vi "AlGaInPAs_prep_run_cont_dil_v17.vi"(2 "Debug Mode":bool, 3 "Elapsed Time(s)":dbl, 4 "State":enum16{"Edit", "Start", "Run", "End", "Idle"}(ring), 5 "Argument List In":string[](array[string])) -> (0 "Status Out":string, 1 "Argument List Out":string[](array[string]))   [LabVIEW 2011]
panel:
  out "GAMFC3 var":dbl=100.0 caption="R3 (0-1000 sscm)" format="%.1f"
  out "GAMFC2 var":dbl=10.0 caption="R2 (0-100 sscm)" format="%.2f"
  out "GAMFC1 var":dbl=1.0 caption="R1 (0-10 sscm)" format="%.2f"
  out "Ga Flow var":dbl=1.0 caption="Ga Flow (0-10 sscm)" format="%.4f"
  out "Prep-In var":bool
  out "Prep-Ga var":bool
  out "Prep-Al var":bool
  out "Prep-P var":bool
  out "Prep-As var":bool
  out "prep_done":bool
  out "run started":bool
  out "first":bool=TRUE
  out "total time":dbl
  out "is OK?":bool
  out "AsH3?":bool
  out "PH3?":bool
  out "In?":bool
  out "Ga?":bool
  out "Al?":bool
  in  "Prep As":bool caption="Pre-run"
  in  "Prep P":bool caption="Pre-run"
  in  "Prep In":bool caption="Pre-run"
  in  "prep_time":dbl caption="pre-run time (s)"
  in  "Prep Al":bool caption="Pre-run"
  in  "Run As":bool caption="Run"
  in  "AsH3 Flow":dbl caption="AsH3 Flow (0-10 sccm)" format="%.2f"
  in  "P Flow":dbl caption="P Flow (0-100 sccm)" format="%.2f"
  in  "Run P":bool caption="Run"
  in  "In Flow":dbl caption="In Flow (0-100 sscm)" format="%.2f"
  in  "Run In":bool caption="Run"
  in  "Run Al":bool caption="Run"
  in  "Al Flow":dbl caption="Al Flow (0-100 sscm)" format="%.2f"
  in  "Cancel":bool
  in  "OK":bool
  out "tTotal(s) 2":dbl
  in  "Ga Tab Control":enum32{"Page 1", "Page 2", "Page 3"}(tab)
  in  "Ga Dilution":bool caption="Dilute"
  in  "Run Ga":bool caption="Run"
  in  "Prep Ga":bool caption="Pre-run"
  out "Ga Flow val":dbl=1.0 caption="Ga Flow (0-10 sscm)" format="%.4f"
  in  "Ga Flow set":dbl=1.0 caption="Ga Flow (0-10 sscm)" format="%.4f"
  out "GAMFC1 val":dbl=1.0 caption="R1 (0-10 sscm)" format="%.4f"
  out "GAMFC3 val":dbl=100.0 caption="R3 (0-1000 sscm)" format="%.1f"
  out "GAMFC2 val":dbl=10.0 caption="R2 (0-100 sscm)" format="%.2f"
  in  "GAMFC1 set":dbl=1.0 caption="R1 (0-10 sscm)" format="%.2f"
  in  "GAMFC2 set":dbl=10.0 caption="R2 (0-100 sscm)" format="%.2f"
  in  "GAMFC3 set":dbl=100.0 caption="R3 (0-1000 sscm)" format="%.1f"
  in  "Ga Calculated":u16(ring)=1 caption="Calculated" items=["Ga flow", "MFC1", "MFC2", "MFC3"]
  # "Add pre-run time to run time in editor."
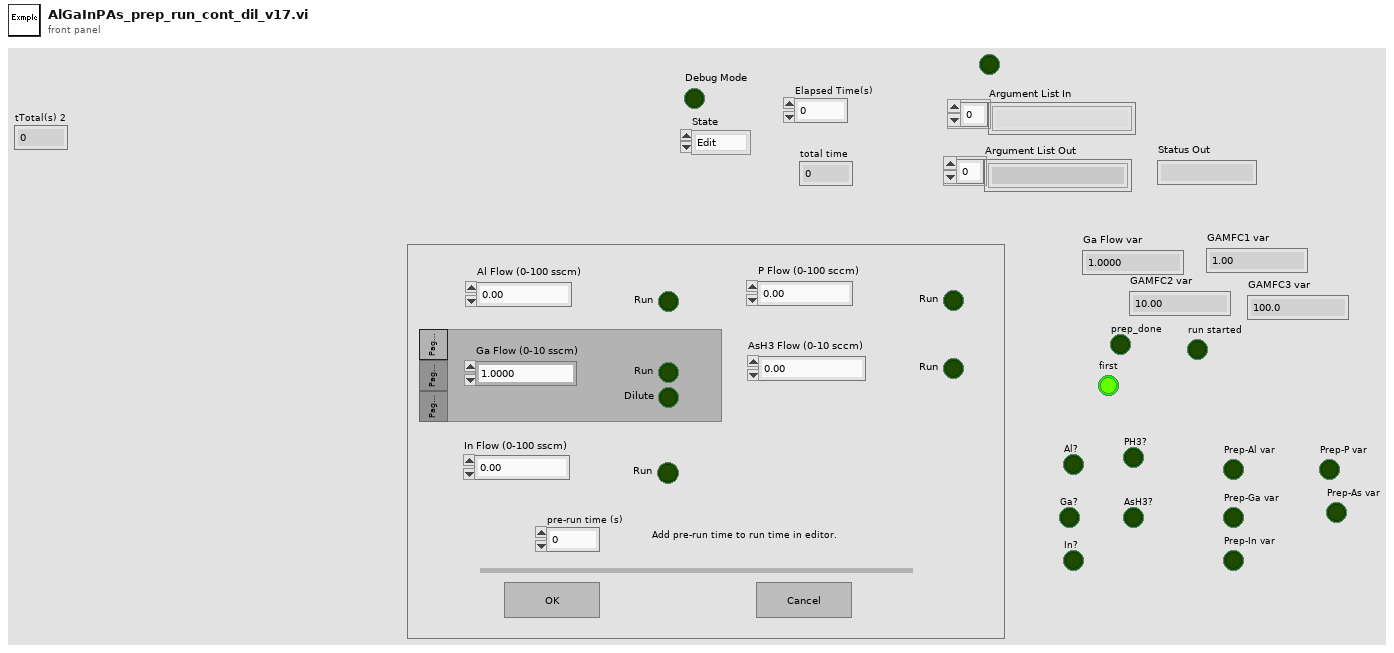
[diagram p1: front panel]
types:
  T1 = enum16{"Discrete", "Continuous", "Instantaneous", "Finite"}
  T2 = enum32{"Invalid", "Default", "Floating", "Floating/Auto-Hide", "Modal"}
  T3 = cluster{"Ga val":bool, "MFC1 val":bool, "MFC2 val":bool, "MFC3 val":bool, "Ga set":bool, "MFC1 set":bool, "MFC2 set":bool, "MFC3 set":bool}
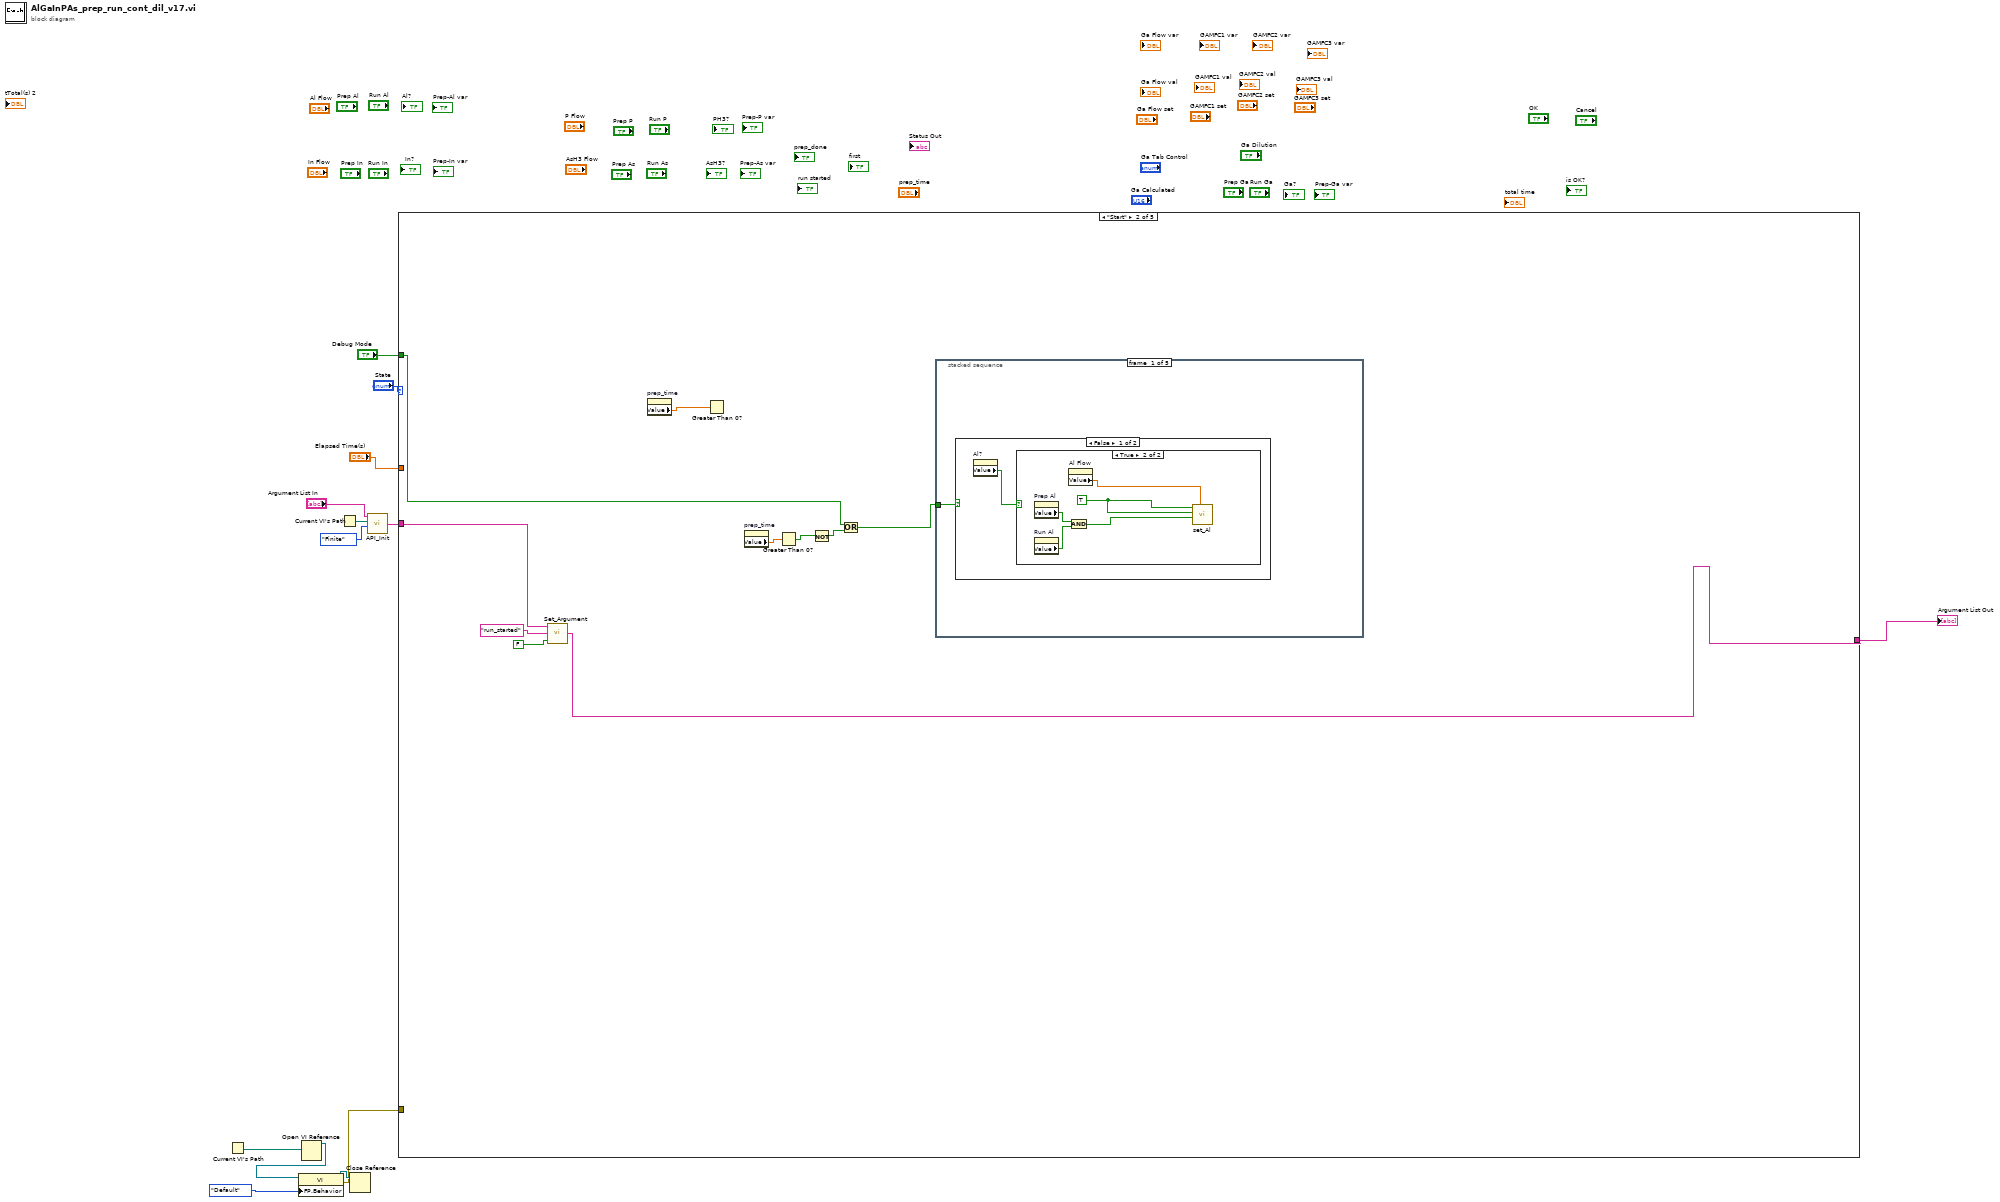
[diagram p0: block diagram]
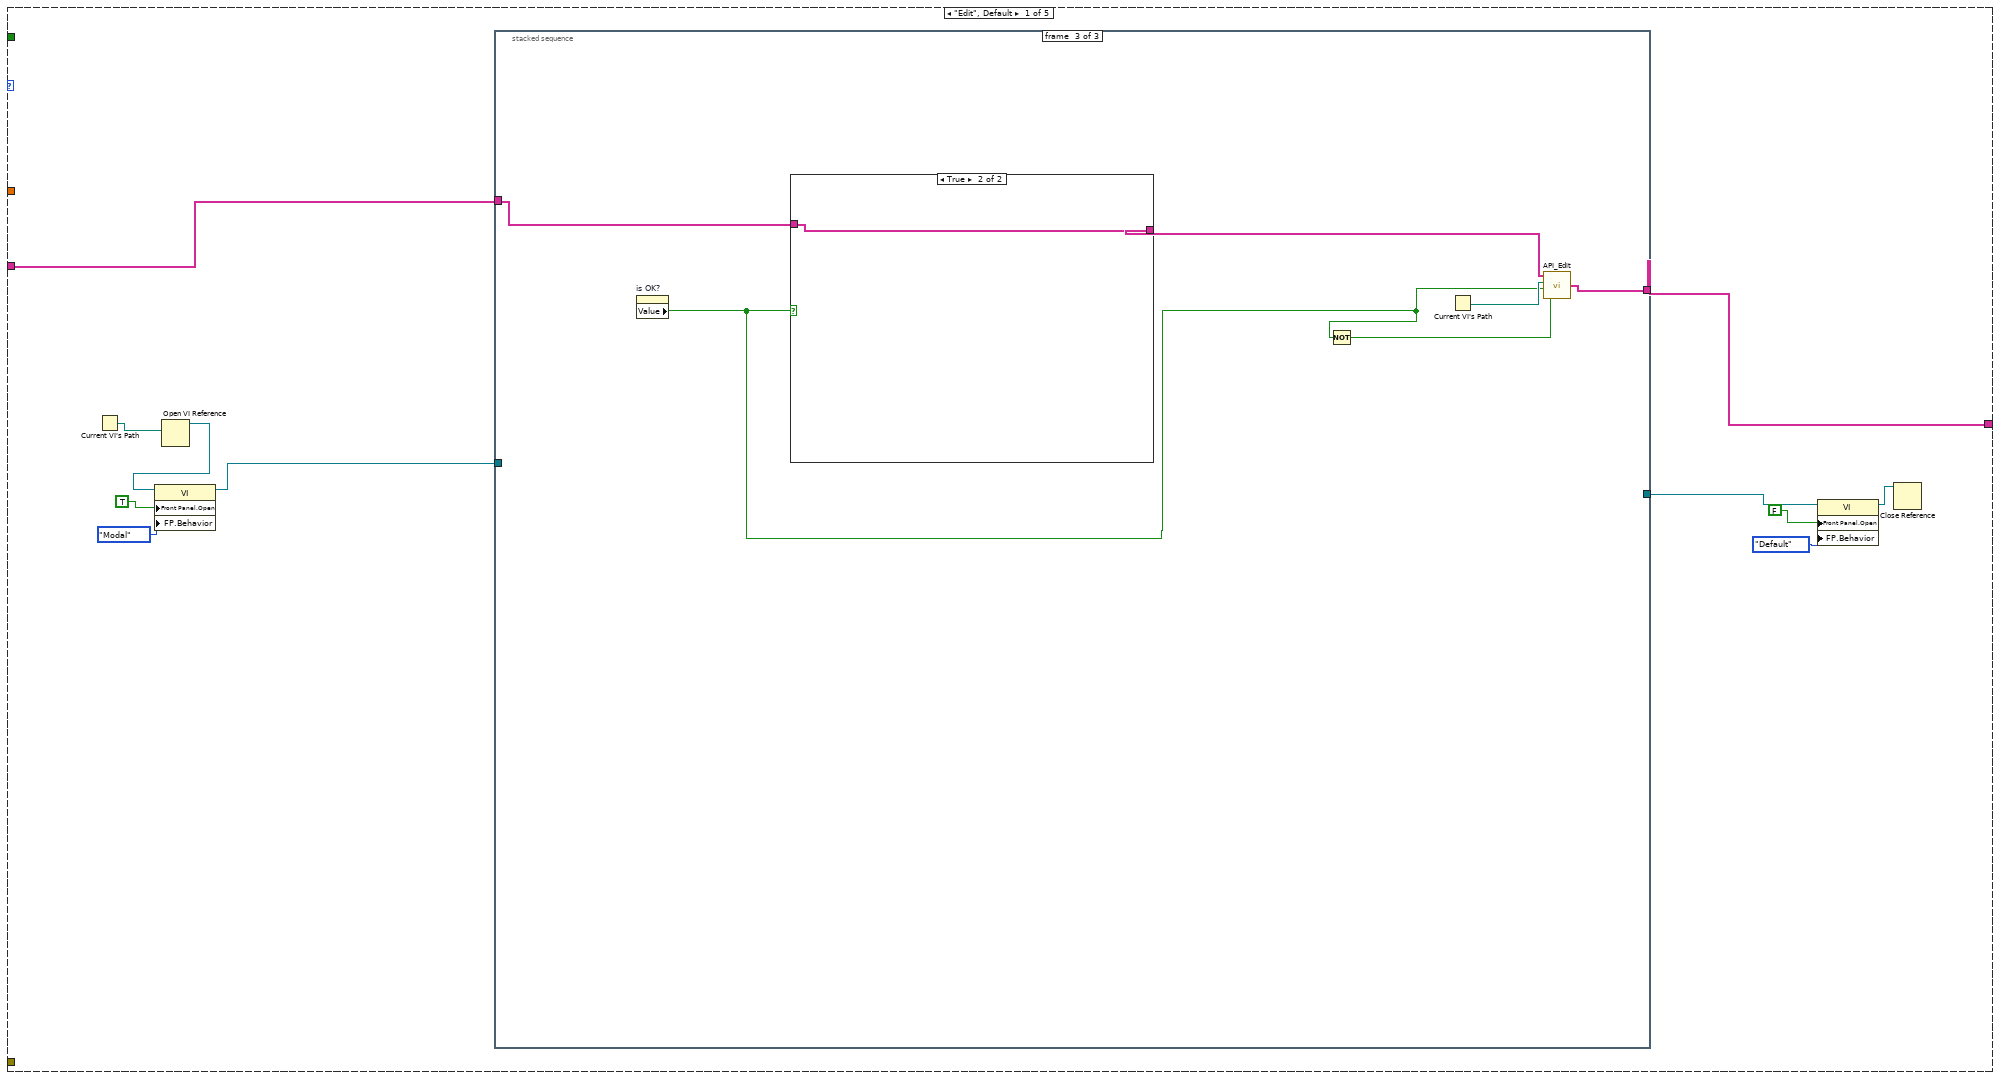
[diagram p2: hidden frame]
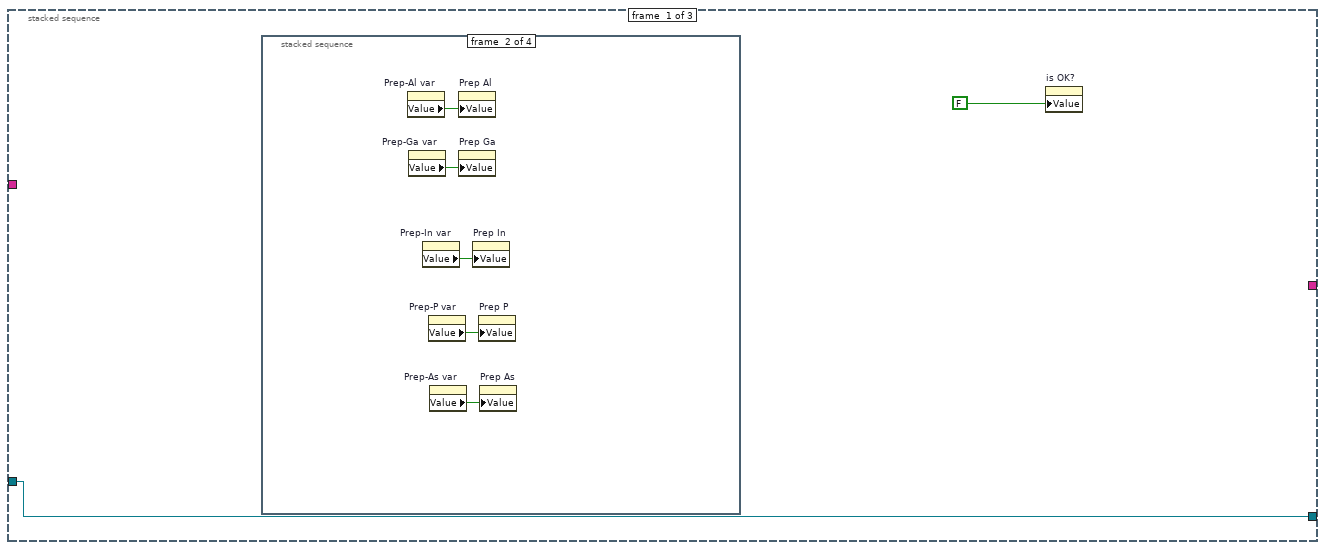
[diagram p3: hidden frame]
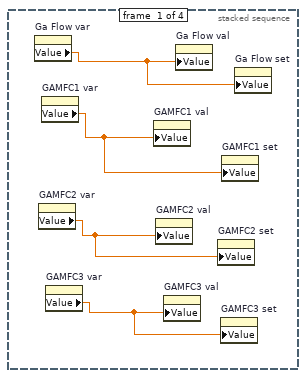
[diagram p4: hidden frame]
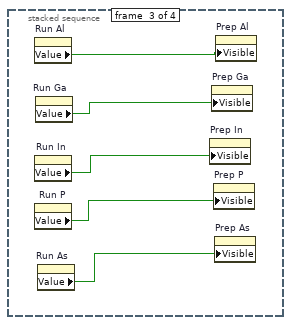
[diagram p5: hidden frame]
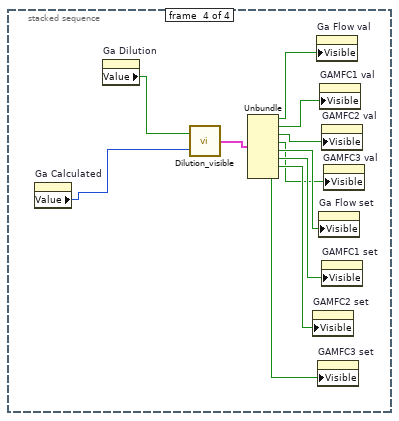
[diagram p6: hidden frame]
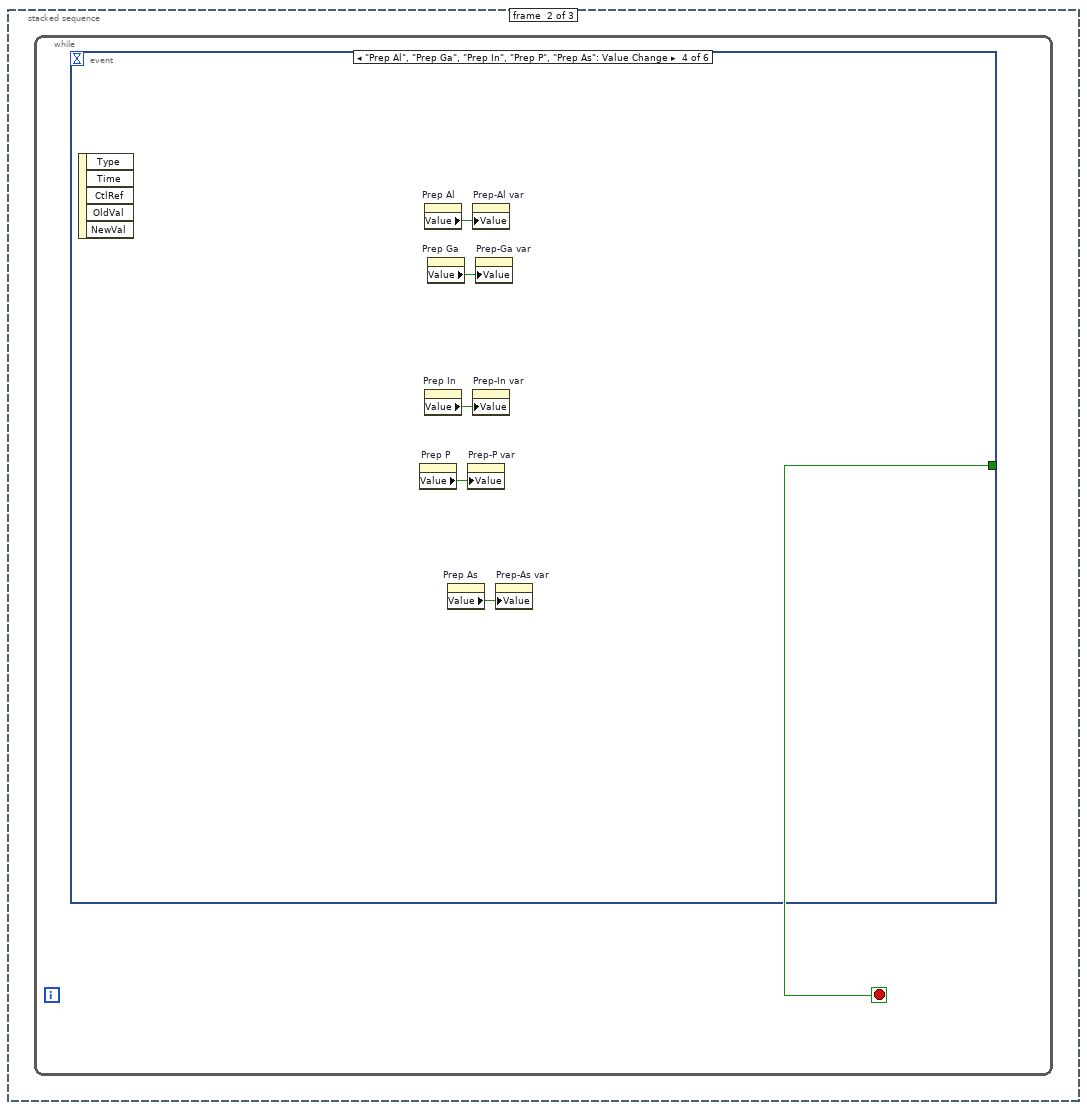
[diagram p7: hidden frame]
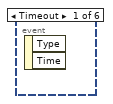
[diagram p8: hidden frame]
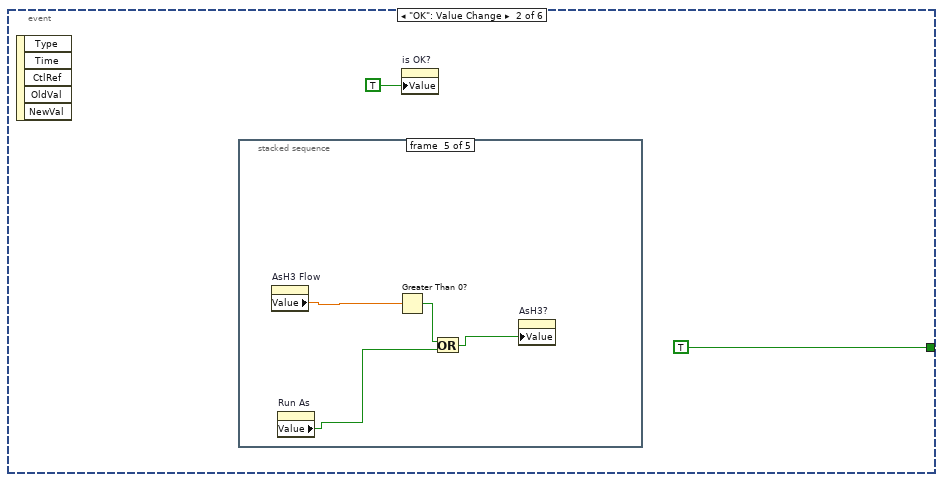
[diagram p9: hidden frame]
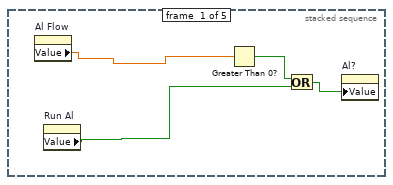
[diagram p10: hidden frame]
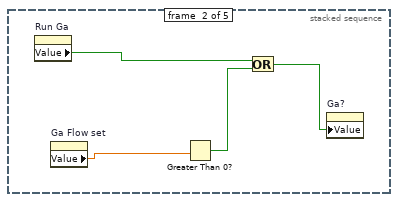
[diagram p11: hidden frame]
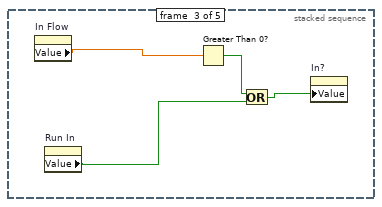
[diagram p12: hidden frame]
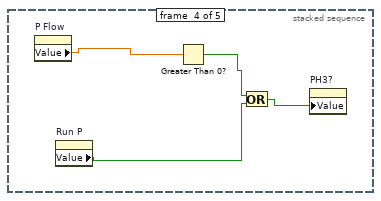
[diagram p13: hidden frame]
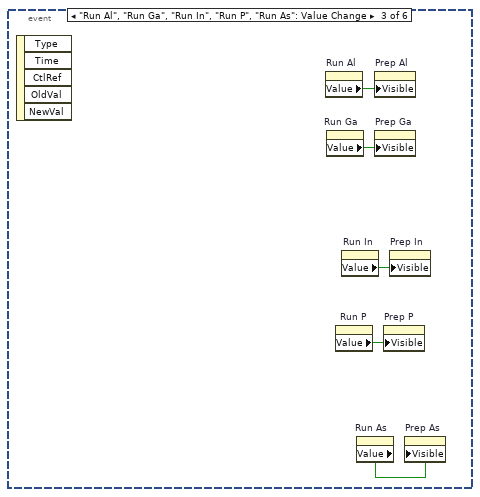
[diagram p14: hidden frame]
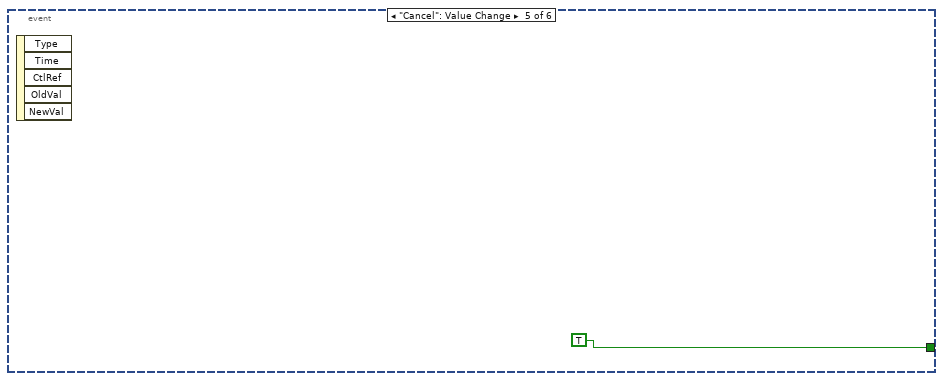
[diagram p15: hidden frame]
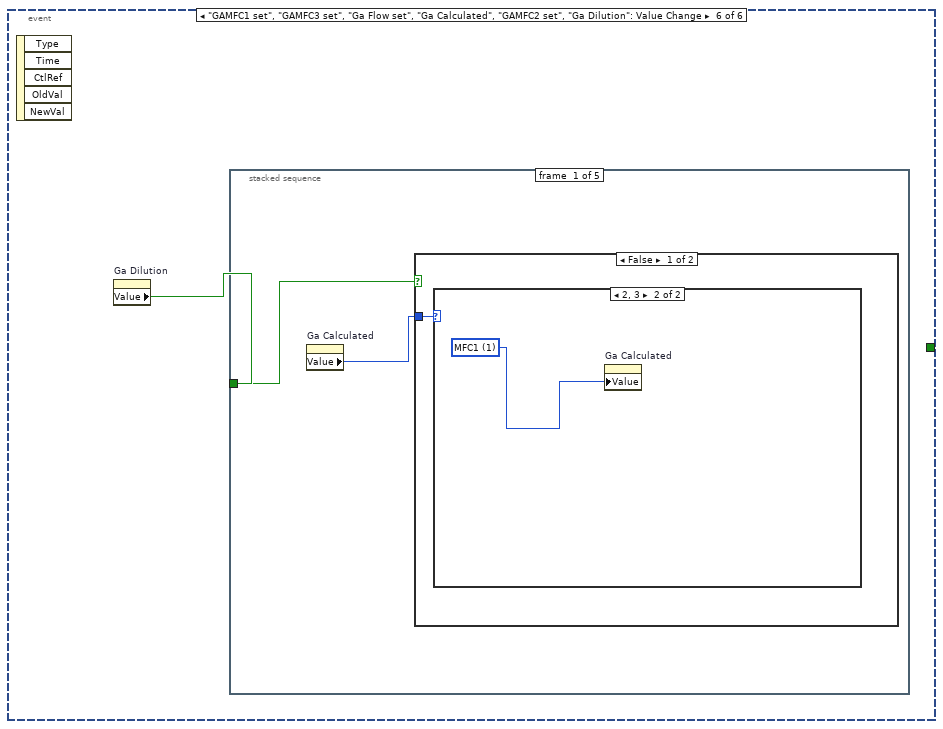
[diagram p16: hidden frame]
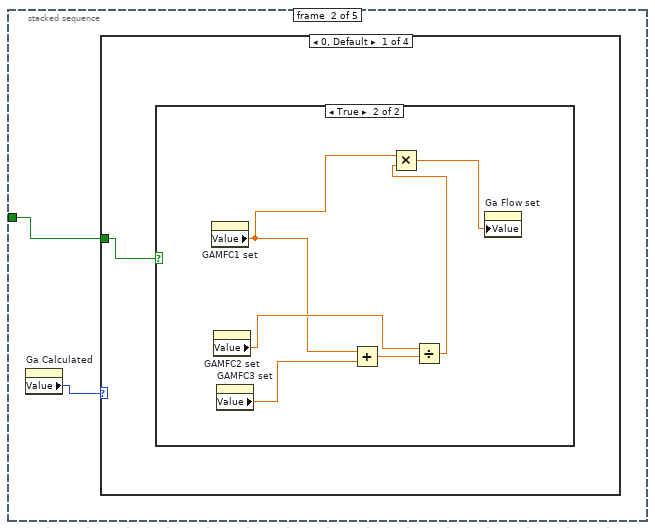
[diagram p19: hidden frame]
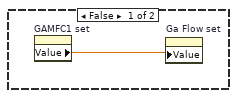
[diagram p20: hidden frame]
diagram:
  n1 = Current VI's Path() -> (path=w9:path)
  n2 = Open VI Reference(vi path=w9) -> (vi reference=w8:refnum<vi>)  [unwired: 1 in, 5 out]
  n3 = property class="VI"(reference=w8, "FP.Behavior"=T2."Default" ("Front Panel Window:Behavior")) -> (reference out=w6:refnum<vi>, error out=w5:errorcluster)  [unwired: 1 in]
  n4 = Current VI's Path() -> (path=w4:path)
  n5 = Close Reference(reference=w6) -> ()  [unwired: 1 in, 1 out]
  n6 = call "API_Init.vi"("API Mode"=T1."Finite", "VI Path"=w4, "Argument List In"="Argument List In") -> ("Argument List Out"=w1:string[])  [unwired: 1 in]
  n7 = case shown="\"Start\"" "State" {
    tunnel: "Debug Mode" -> [_ w149 w208 _ _]
    tunnel: "Elapsed Time(s)" -> [_ _ w210 _ _]
    tunnel: w1 -> [w15 w156 w207 w325 w326]
    tunnel: [w14 w155 w209 w325 w326] -> w10
    tunnel: w5 -> [_ _ _ _ _]
    frame "Edit", Default {
      n8 = Current VI's Path() -> (path=w20:path)
      n9 = Open VI Reference(vi path=w20) -> (vi reference=w19:refnum<vi>)  [unwired: 1 in, 5 out]
      n10 = property class="VI"(reference=w19, "Front Panel.Open"=TRUE ("Front Panel Window:Open"), "FP.Behavior"=T2."Modal" ("Front Panel Window:Behavior")) -> (reference out=w18:refnum<vi>)  [unwired: 1 in, 1 out]
      n11 = stacked-sequence {
        tunnel: w15 -> [_ _ w144]
        tunnel: w18 -> [w26 _ _]
        tunnel: [w26 _ _] -> w22
        tunnel: [_ _ w142] -> w14
        frame #0 {
          n12 = stacked-sequence {
            frame #0 {
              n13 = property on="Ga Flow var" class="DigNum (strict)"() -> ("Value"=w30:dbl)  [unwired: 2 in, 2 out]
              n14 = property on="GAMFC2 var" class="DigNum (strict)"() -> ("Value"=w28:dbl)  [unwired: 2 in, 2 out]
              n15 = property on="GAMFC1 var" class="DigNum (strict)"() -> ("Value"=w27:dbl)  [unwired: 2 in, 2 out]
              n16 = property on="GAMFC3 var" class="DigNum (strict)"() -> ("Value"=w29:dbl)  [unwired: 2 in, 2 out]
              n17 = property on="GAMFC1 val" class="DigNum (strict)"("Value"=w27) -> ()  [unwired: 2 in, 2 out]
              n18 = property on="GAMFC2 val" class="DigNum (strict)"("Value"=w28) -> ()  [unwired: 2 in, 2 out]
              n19 = property on="GAMFC3 val" class="DigNum (strict)"("Value"=w29) -> ()  [unwired: 2 in, 2 out]
              n20 = property on="Ga Flow val" class="DigNum (strict)"("Value"=w30) -> ()  [unwired: 2 in, 2 out]
              n21 = property on="GAMFC2 set" class="DigNum (strict)"("Value"=w28) -> ()  [unwired: 2 in, 2 out]
              n22 = property on="GAMFC3 set" class="DigNum (strict)"("Value"=w29) -> ()  [unwired: 2 in, 2 out]
              n23 = property on="GAMFC1 set" class="DigNum (strict)"("Value"=w27) -> ()  [unwired: 2 in, 2 out]
              n24 = property on="Ga Flow set" class="DigNum (strict)"("Value"=w30) -> ()  [unwired: 2 in, 2 out]
            }
            frame #1 {
              n25 = property on="Prep-Al var" class="Bool (strict)"() -> ("Value"=w35:bool)  [unwired: 2 in, 2 out]
              n26 = property on="Prep-Ga var" class="Bool (strict)"() -> ("Value"=w34:bool)  [unwired: 2 in, 2 out]
              n27 = property on="Prep-In var" class="Bool (strict)"() -> ("Value"=w33:bool)  [unwired: 2 in, 2 out]
              n28 = property on="Prep-P var" class="Bool (strict)"() -> ("Value"=w32:bool)  [unwired: 2 in, 2 out]
              n29 = property on="Prep-As var" class="Bool (strict)"() -> ("Value"=w31:bool)  [unwired: 2 in, 2 out]
              n30 = property on="Prep Al" class="Bool (strict)"("Value"=w35) -> ()  [unwired: 2 in, 2 out]
              n31 = property on="Prep Ga" class="Bool (strict)"("Value"=w34) -> ()  [unwired: 2 in, 2 out]
              n32 = property on="Prep In" class="Bool (strict)"("Value"=w33) -> ()  [unwired: 2 in, 2 out]
              n33 = property on="Prep P" class="Bool (strict)"("Value"=w32) -> ()  [unwired: 2 in, 2 out]
              n34 = property on="Prep As" class="Bool (strict)"("Value"=w31) -> ()  [unwired: 2 in, 2 out]
            }
            frame #2 {
              n35 = property on="Run Al" class="Bool (strict)"() -> ("Value"=w40:bool)  [unwired: 2 in, 2 out]
              n36 = property on="Run In" class="Bool (strict)"() -> ("Value"=w38:bool)  [unwired: 2 in, 2 out]
              n37 = property on="Run P" class="Bool (strict)"() -> ("Value"=w37:bool)  [unwired: 2 in, 2 out]
              n38 = property on="Run Ga" class="Bool (strict)"() -> ("Value"=w39:bool)  [unwired: 2 in, 2 out]
              n39 = property on="Run As" class="Bool (strict)"() -> ("Value"=w36:bool)  [unwired: 2 in, 2 out]
              n40 = property on="Prep In" class="Bool (strict)"("Visible"=w38) -> ()  [unwired: 2 in, 2 out]
              n41 = property on="Prep Ga" class="Bool (strict)"("Visible"=w39) -> ()  [unwired: 2 in, 2 out]
              n42 = property on="Prep P" class="Bool (strict)"("Visible"=w37) -> ()  [unwired: 2 in, 2 out]
              n43 = property on="Prep As" class="Bool (strict)"("Visible"=w36) -> ()  [unwired: 2 in, 2 out]
              n44 = property on="Prep Al" class="Bool (strict)"("Visible"=w40) -> ()  [unwired: 2 in, 2 out]
            }
            frame #3 {
              n45 = property on="Ga Calculated" class="Ring (strict)"() -> ("Value"=w41:u16)  [unwired: 2 in, 2 out]
              n46 = property on="Ga Dilution" class="Bool (strict)"() -> ("Value"=w51:bool)  [unwired: 2 in, 2 out]
              n47 = call "Dilution_visible.vi"("calculated"=w41, "dilution"=w51) -> ("Visible"=w43:T3)
              n48 = Unbundle(w43) -> ("Ga val"=w44:bool, "MFC1 val"=w45:bool, "MFC2 val"=w42:bool, "MFC3 val"=w46:bool, "Ga set"=w47:bool, "MFC1 set"=w48:bool, "MFC2 set"=w49:bool, "MFC3 set"=w50:bool)
              n49 = property on="GAMFC2 set" class="DigNum (strict)"("Visible"=w49) -> ()  [unwired: 2 in, 2 out]
              n50 = property on="Ga Flow val" class="DigNum (strict)"("Visible"=w44) -> ()  [unwired: 2 in, 2 out]
              n51 = property on="GAMFC3 set" class="DigNum (strict)"("Visible"=w50) -> ()  [unwired: 2 in, 2 out]
              n52 = property on="Ga Flow set" class="DigNum (strict)"("Visible"=w47) -> ()  [unwired: 2 in, 2 out]
              n53 = property on="GAMFC1 val" class="DigNum (strict)"("Visible"=w45) -> ()  [unwired: 2 in, 2 out]
              n54 = property on="GAMFC2 val" class="DigNum (strict)"("Visible"=w42) -> ()  [unwired: 2 in, 2 out]
              n55 = property on="GAMFC1 set" class="DigNum (strict)"("Visible"=w48) -> ()  [unwired: 2 in, 2 out]
              n56 = property on="GAMFC3 val" class="DigNum (strict)"("Visible"=w46) -> ()  [unwired: 2 in, 2 out]
            }
          }
          n57 = property on="is OK?" class="Bool (strict)"("Value"=FALSE ("is OK?")) -> ()  [unwired: 2 in, 2 out]
        }
        frame #1 {
          n58 = while {
            stop <- w52 stop-if-true
            n59 = event shown="[3] \"Prep Al\", \"Prep Ga\", \"Prep In\", \"Prep P\", \"Prep As\": Value Change" {
              selector: _ -> [_ _ _ _ _ _]
              dyn-events: _ -> [_ _ _ _ _ _]
              timeout: _ -> [_ _ _ _ _ _]
              tunnel: [_ TRUE _ _ TRUE _] -> w52
              event Timeout {
                n60 = event-data() -> ()  [unwired: 1 in, 2 out]
              }
              event "OK": Value Change {
                n61 = event-data() -> ()  [unwired: 1 in, 5 out]
                n62 = stacked-sequence {
                  frame #0 {
                    n63 = property on="Al Flow" class="DigNum (strict)"() -> ("Value"=w57:dbl)  [unwired: 2 in, 2 out]
                    n64 = property on="Run Al" class="Bool (strict)"() -> ("Value"=w56:bool)  [unwired: 2 in, 2 out]
                    n65 = Greater Than 0?(x=w57) -> (x > 0?=w58:bool)
                    n66 = Or(x=w58, y=w56) -> (x .or. y?=w55:bool)
                    n67 = property on="Al?" class="Bool (strict)"("Value"=w55) -> ()  [unwired: 2 in, 2 out]
                  }
                  frame #1 {
                    n68 = property on="Run Ga" class="Bool (strict)"() -> ("Value"=w60:bool)  [unwired: 2 in, 2 out]
                    n69 = property on="Ga Flow set" class="DigNum (strict)"() -> ("Value"=w61:dbl)  [unwired: 2 in, 2 out]
                    n70 = Greater Than 0?(x=w61) -> (x > 0?=w62:bool)
                    n71 = Or(x=w60, y=w62) -> (x .or. y?=w59:bool)
                    n72 = property on="Ga?" class="Bool (strict)"("Value"=w59) -> ()  [unwired: 2 in, 2 out]
                  }
                  frame #2 {
                    n73 = property on="In Flow" class="DigNum (strict)"() -> ("Value"=w64:dbl)  [unwired: 2 in, 2 out]
                    n74 = property on="Run In" class="Bool (strict)"() -> ("Value"=w65:bool)  [unwired: 2 in, 2 out]
                    n75 = Greater Than 0?(x=w64) -> (x > 0?=w66:bool)
                    n76 = Or(x=w66, y=w65) -> (x .or. y?=w63:bool)
                    n77 = property on="In?" class="Bool (strict)"("Value"=w63) -> ()  [unwired: 2 in, 2 out]
                  }
                  frame #3 {
                    n78 = property on="P Flow" class="DigNum (strict)"() -> ("Value"=w69:dbl)  [unwired: 2 in, 2 out]
                    n79 = property on="Run P" class="Bool (strict)"() -> ("Value"=w68:bool)  [unwired: 2 in, 2 out]
                    n80 = Greater Than 0?(x=w69) -> (x > 0?=w70:bool)
                    n81 = Or(x=w70, y=w68) -> (x .or. y?=w67:bool)
                    n82 = property on="PH3?" class="Bool (strict)"("Value"=w67) -> ()  [unwired: 2 in, 2 out]
                  }
                  frame #4 {
                    n83 = property on="AsH3 Flow" class="DigNum (strict)"() -> ("Value"=w73:dbl)  [unwired: 2 in, 2 out]
                    n84 = property on="Run As" class="Bool (strict)"() -> ("Value"=w72:bool)  [unwired: 2 in, 2 out]
                    n85 = Greater Than 0?(x=w73) -> (x > 0?=w74:bool)
                    n86 = Or(x=w74, y=w72) -> (x .or. y?=w71:bool)
                    n87 = property on="AsH3?" class="Bool (strict)"("Value"=w71) -> ()  [unwired: 2 in, 2 out]
                  }
                }
                n88 = property on="is OK?" class="Bool (strict)"("Value"=TRUE ("is OK?")) -> ()  [unwired: 2 in, 2 out]
              }
              event "Run Al", "Run Ga", "Run In", "Run P", "Run As": Value Change {
                n89 = event-data() -> ()  [unwired: 1 in, 5 out]
                n90 = property on="Run Al" class="Bool (strict)"() -> ("Value"=w79:bool)  [unwired: 2 in, 2 out]
                n91 = property on="Run Ga" class="Bool (strict)"() -> ("Value"=w78:bool)  [unwired: 2 in, 2 out]
                n92 = property on="Run P" class="Bool (strict)"() -> ("Value"=w75:bool)  [unwired: 2 in, 2 out]
                n93 = property on="Run In" class="Bool (strict)"() -> ("Value"=w77:bool)  [unwired: 2 in, 2 out]
                n94 = property on="Run As" class="Bool (strict)"() -> ("Value"=w76:bool)  [unwired: 2 in, 2 out]
                n95 = property on="Prep Al" class="Bool (strict)"("Visible"=w79) -> ()  [unwired: 2 in, 2 out]
                n96 = property on="Prep Ga" class="Bool (strict)"("Visible"=w78) -> ()  [unwired: 2 in, 2 out]
                n97 = property on="Prep P" class="Bool (strict)"("Visible"=w75) -> ()  [unwired: 2 in, 2 out]
                n98 = property on="Prep In" class="Bool (strict)"("Visible"=w77) -> ()  [unwired: 2 in, 2 out]
                n99 = property on="Prep As" class="Bool (strict)"("Visible"=w76) -> ()  [unwired: 2 in, 2 out]
              }
              event "Prep Al", "Prep Ga", "Prep In", "Prep P", "Prep As": Value Change {
                n100 = event-data() -> ()  [unwired: 1 in, 5 out]
                n101 = property on="Prep P" class="Bool (strict)"() -> ("Value"=w81:bool)  [unwired: 2 in, 2 out]
                n102 = property on="Prep Al" class="Bool (strict)"() -> ("Value"=w84:bool)  [unwired: 2 in, 2 out]
                n103 = property on="Prep In" class="Bool (strict)"() -> ("Value"=w82:bool)  [unwired: 2 in, 2 out]
                n104 = property on="Prep Ga" class="Bool (strict)"() -> ("Value"=w83:bool)  [unwired: 2 in, 2 out]
                n105 = property on="Prep As" class="Bool (strict)"() -> ("Value"=w80:bool)  [unwired: 2 in, 2 out]
                n106 = property on="Prep-P var" class="Bool (strict)"("Value"=w81) -> ()  [unwired: 2 in, 2 out]
                n107 = property on="Prep-Al var" class="Bool (strict)"("Value"=w84) -> ()  [unwired: 2 in, 2 out]
                n108 = property on="Prep-In var" class="Bool (strict)"("Value"=w82) -> ()  [unwired: 2 in, 2 out]
                n109 = property on="Prep-Ga var" class="Bool (strict)"("Value"=w83) -> ()  [unwired: 2 in, 2 out]
                n110 = property on="Prep-As var" class="Bool (strict)"("Value"=w80) -> ()  [unwired: 2 in, 2 out]
              }
              event "Cancel": Value Change {
                n111 = event-data() -> ()  [unwired: 1 in, 5 out]
              }
              event "GAMFC1 set", "GAMFC3 set", "Ga Flow set", "Ga Calculated", "GAMFC2 set", "Ga Dilution": Value Change {
                n112 = event-data() -> ()  [unwired: 1 in, 5 out]
                n113 = property on="Ga Dilution" class="Bool (strict)"() -> ("Value"=w86:bool)  [unwired: 2 in, 2 out]
                n114 = stacked-sequence {
                  tunnel: w86 -> [w88 w92 w133 _ w138]
                  frame #0 {
                    n115 = property on="Ga Calculated" class="Ring (strict)"() -> ("Value"=w87:u16)  [unwired: 2 in, 2 out]
                    n116 = case shown="False" w88 {
                      tunnel: w87 -> [w89 _]
                      frame False {
                        n117 = case shown="2, 3" w89 {
                          frame 0, 1, Default {
                          }
                          frame 2, 3 {
                            w90 = u16 1 items=["Ga flow", "MFC1", "MFC2", "MFC3"] ("Ga calculated")
                            n118 = property on="Ga Calculated" class="Ring (strict)"("Value"=w90) -> ()  [unwired: 2 in, 2 out]
                          }
                        }
                      }
                      frame True {
                      }
                    }
                  }
                  frame #1 {
                    n119 = property on="Ga Calculated" class="Ring (strict)"() -> ("Value"=w91:u16)  [unwired: 2 in, 2 out]
                    n120 = case shown="0, Default" w91 {
                      tunnel: w92 -> [w93 w101 w109 w116]
                      frame 0, Default {
                        n121 = case shown="True" w93 {
                          frame False {
                            n122 = property on="GAMFC1 set" class="DigNum (strict)"() -> ("Value"=w94:dbl)  [unwired: 2 in, 2 out]
                            n123 = property on="Ga Flow set" class="DigNum (strict)"("Value"=w94) -> ()  [unwired: 2 in, 2 out]
                          }
                          frame True {
                            n124 = property on="GAMFC1 set" class="DigNum (strict)"() -> ("Value"=w96:dbl)  [unwired: 2 in, 2 out]
                            n125 = property on="GAMFC2 set" class="DigNum (strict)"() -> ("Value"=w98:dbl)  [unwired: 2 in, 2 out]
                            n126 = property on="GAMFC3 set" class="DigNum (strict)"() -> ("Value"=w100:dbl)  [unwired: 2 in, 2 out]
                            n127 = Add(x=w96, y=w100) -> (x+y=w99:dbl)
                            n128 = Divide(x=w98, y=w99) -> (x/y=w97:dbl)
                            n129 = Multiply(x=w96, y=w97) -> (x*y=w95:dbl)
                            n130 = property on="Ga Flow set" class="DigNum (strict)"("Value"=w95) -> ()  [unwired: 2 in, 2 out]
                          }
                        }
                      }
                      frame 1 {
                        n131 = case shown="True" w101 {
                          frame False {
                            n132 = property on="Ga Flow set" class="DigNum (strict)"() -> ("Value"=w102:dbl)  [unwired: 2 in, 2 out]
                            n133 = property on="GAMFC1 set" class="DigNum (strict)"("Value"=w102) -> ()  [unwired: 2 in, 2 out]
                          }
                          frame True {
                            n134 = property on="Ga Flow set" class="DigNum (strict)"() -> ("Value"=w107:dbl)  [unwired: 2 in, 2 out]
                            n135 = property on="GAMFC2 set" class="DigNum (strict)"() -> ("Value"=w108:dbl)  [unwired: 2 in, 2 out]
                            n136 = property on="GAMFC3 set" class="DigNum (strict)"() -> ("Value"=w106:dbl)  [unwired: 2 in, 2 out]
                            n137 = Subtract(x=w108, y=w107) -> (x-y=w104:dbl)
                            n138 = Multiply(x=w107, y=w106) -> (x*y=w105:dbl)
                            n139 = Divide(x=w105, y=w104) -> (x/y=w103:dbl)
                            n140 = property on="GAMFC1 set" class="DigNum (strict)"("Value"=w103) -> ()  [unwired: 2 in, 2 out]
                          }
                        }
                      }
                      frame 2 {
                        n141 = case shown="True" w109 {
                          frame False {
                          }
                          frame True {
                            n142 = property on="GAMFC1 set" class="DigNum (strict)"() -> ("Value"=w111:dbl)  [unwired: 2 in, 2 out]
                            n143 = property on="GAMFC3 set" class="DigNum (strict)"() -> ("Value"=w113:dbl)  [unwired: 2 in, 2 out]
                            n144 = property on="Ga Flow set" class="DigNum (strict)"() -> ("Value"=w114:dbl)  [unwired: 2 in, 2 out]
                            n145 = Add(x=w111, y=w113) -> (x+y=w115:dbl)
                            n146 = Multiply(x=w114, y=w115) -> (x*y=w112:dbl)
                            n147 = Divide(x=w112, y=w111) -> (x/y=w110:dbl)
                            n148 = property on="GAMFC2 set" class="DigNum (strict)"("Value"=w110) -> ()  [unwired: 2 in, 2 out]
                          }
                        }
                      }
                      frame 3 {
                        n149 = case shown="True" w116 {
                          frame False {
                          }
                          frame True {
                            n150 = property on="GAMFC2 set" class="DigNum (strict)"() -> ("Value"=w122:dbl)  [unwired: 2 in, 2 out]
                            n151 = property on="Ga Flow set" class="DigNum (strict)"() -> ("Value"=w120:dbl)  [unwired: 2 in, 2 out]
                            n152 = property on="GAMFC1 set" class="DigNum (strict)"() -> ("Value"=w121:dbl)  [unwired: 2 in, 2 out]
                            n153 = Subtract(x=w122, y=w120) -> (x-y=w118:dbl)
                            n154 = Divide(x=w121, y=w120) -> (x/y=w119:dbl)
                            n155 = Multiply(x=w119, y=w118) -> (x*y=w117:dbl)
                            n156 = property on="GAMFC3 set" class="DigNum (strict)"("Value"=w117) -> ()  [unwired: 2 in, 2 out]
                          }
                        }
                      }
                    }
                  }
                  frame #2 {
                    n157 = property on="Ga Calculated" class="Ring (strict)"() -> ("Value"=w123:u16)  [unwired: 2 in, 2 out]
                    n158 = call "Dilution_visible.vi"("calculated"=w123, "dilution"=w133) -> ("Visible"=w129:T3)
                    n159 = Unbundle(w129) -> ("Ga val"=w132:bool, "MFC1 val"=w131:bool, "MFC2 val"=w130:bool, "MFC3 val"=w128:bool, "Ga set"=w127:bool, "MFC1 set"=w126:bool, "MFC2 set"=w125:bool, "MFC3 set"=w124:bool)
                    n160 = property on="Ga Flow set" class="DigNum (strict)"("Visible"=w127) -> ()  [unwired: 2 in, 2 out]
                    n161 = property on="GAMFC1 set" class="DigNum (strict)"("Visible"=w126) -> ()  [unwired: 2 in, 2 out]
                    n162 = property on="GAMFC3 set" class="DigNum (strict)"("Visible"=w124) -> ()  [unwired: 2 in, 2 out]
                    n163 = property on="GAMFC2 set" class="DigNum (strict)"("Visible"=w125) -> ()  [unwired: 2 in, 2 out]
                    n164 = property on="Ga Flow val" class="DigNum (strict)"("Visible"=w132) -> ()  [unwired: 2 in, 2 out]
                    n165 = property on="GAMFC1 val" class="DigNum (strict)"("Visible"=w131) -> ()  [unwired: 2 in, 2 out]
                    n166 = property on="GAMFC2 val" class="DigNum (strict)"("Visible"=w130) -> ()  [unwired: 2 in, 2 out]
                    n167 = property on="GAMFC3 val" class="DigNum (strict)"("Visible"=w128) -> ()  [unwired: 2 in, 2 out]
                  }
                  frame #3 {
                    n168 = property on="GAMFC1 set" class="DigNum (strict)"() -> ("Value"=w136:dbl)  [unwired: 2 in, 2 out]
                    n169 = property on="Ga Flow set" class="DigNum (strict)"() -> ("Value"=w137:dbl)  [unwired: 2 in, 2 out]
                    n170 = property on="GAMFC2 set" class="DigNum (strict)"() -> ("Value"=w135:dbl)  [unwired: 2 in, 2 out]
                    n171 = property on="GAMFC3 set" class="DigNum (strict)"() -> ("Value"=w134:dbl)  [unwired: 2 in, 2 out]
                    n172 = property on="GAMFC3 val" class="DigNum (strict)"("Value"=w134) -> ()  [unwired: 2 in, 2 out]
                    n173 = property on="GAMFC1 val" class="DigNum (strict)"("Value"=w136) -> ()  [unwired: 2 in, 2 out]
                    n174 = property on="GAMFC2 val" class="DigNum (strict)"("Value"=w135) -> ()  [unwired: 2 in, 2 out]
                    n175 = property on="Ga Flow val" class="DigNum (strict)"("Value"=w137) -> ()  [unwired: 2 in, 2 out]
                    n176 = property on="GAMFC3 var" class="DigNum (strict)"("Value"=w134) -> ()  [unwired: 2 in, 2 out]
                    n177 = property on="GAMFC1 var" class="DigNum (strict)"("Value"=w136) -> ()  [unwired: 2 in, 2 out]
                    n178 = property on="GAMFC2 var" class="DigNum (strict)"("Value"=w135) -> ()  [unwired: 2 in, 2 out]
                    n179 = property on="Ga Flow var" class="DigNum (strict)"("Value"=w137) -> ()  [unwired: 2 in, 2 out]
                  }
                  frame #4 {
                    n180 = case shown="True" w138 {
                      frame False {
                        n181 = property on="Ga Calculated" class="Ring (strict)"("Disabled Items []"=i32[] [2, 3]) -> ()  [unwired: 2 in, 2 out]
                      }
                      frame True {
                        n182 = property on="Ga Calculated" class="Ring (strict)"("Disabled Items []"=i32[] []) -> ()  [unwired: 2 in, 2 out]
                      }
                    }
                  }
                }
              }
            }
          }
        }
        frame #2 {
          n183 = property on="is OK?" class="Bool (strict)"() -> ("Value"=w141:bool)  [unwired: 2 in, 2 out]
          n184 = case shown="True" w141 {
            tunnel: w144 -> [w147 w148]
            tunnel: [w147 w148] -> w143
            frame False {
            }
            frame True {
            }
          }
          n185 = Not(x=w141) -> (.not. x?=w146:bool)
          n186 = Current VI's Path() -> (path=w145:path)
          n187 = call "API_Edit.vi"("Cancel"=w146, "OK"=w141, "VI Path"=w145, "Argument List In"=w143) -> ("Argument List Out"=w142:string[])
        }
      }
      n188 = property class="VI"(reference=w22, "Front Panel.Open"=FALSE ("Front Panel Window:Open"), "FP.Behavior"=T2."Default" ("Front Panel Window:Behavior")) -> (reference out=w23:refnum<vi>)  [unwired: 1 in, 1 out]
      n189 = Close Reference(reference=w23) -> ()  [unwired: 1 in, 1 out]
    }
    frame "Start" {
      n190 = call "Set_Argument.vi"("Enable"=FALSE, "Argument"="run_started", "Argument List In"=w156) -> ("Argument List Out"=w155:string[])
      n191 = property on="prep_time" class="DigNum (strict)"() -> ("Value"=w154:dbl)  [unwired: 2 in, 2 out]
      n192 = Greater Than 0?(x=w154) -> ()  [unwired: 1 out]
      n193 = property on="prep_time" class="DigNum (strict)"() -> ("Value"=w153:dbl)  [unwired: 2 in, 2 out]
      n194 = Greater Than 0?(x=w153) -> (x > 0?=w152:bool)
      n195 = Not(x=w152) -> (.not. x?=w151:bool)
      n196 = Or(x=w149, y=w151) -> (x .or. y?=w150:bool)
      n197 = stacked-sequence {
        tunnel: w150 -> [w159 w168 w180 w189 w198]
        frame #0 {
          n198 = case shown="False" w159 {
            frame False {
              n199 = property on="Al?" class="Bool (strict)"() -> ("Value"=w160:bool)  [unwired: 2 in, 2 out]
              n200 = case shown="True" w160 {
                frame False {
                  w161 = FALSE ("Al Active")
                  n201 = call "set_Al.vi"("ALMFC1"=0.0 ("Aluminum Flow"), "Remote"=w161, "Run"=w161, "Bubbler In"=w161, "Active"=w161) -> ()  [unwired: 5 out]
                }
                frame True {
                  w167 = TRUE ("Al Active")
                  n202 = property on="Prep Al" class="Bool (strict)"() -> ("Value"=w165:bool)  [unwired: 2 in, 2 out]
                  n203 = property on="Run Al" class="Bool (strict)"() -> ("Value"=w164:bool)  [unwired: 2 in, 2 out]
                  n204 = property on="Al Flow" class="DigNum (strict)"() -> ("Value"=w166:dbl)  [unwired: 2 in, 2 out]
                  n205 = And(x=w165, y=w164) -> (x .and. y?=w163:bool)
                  n206 = call "set_Al.vi"("ALMFC1"=w166, "Run"=w163, "Bubbler In"=w167, "Active"=w167) -> ()  [unwired: 1 in, 5 out]
                }
              }
            }
            frame True {
            }
          }
        }
        frame #1 {
          n207 = case shown="False" w168 {
            frame False {
              n208 = property on="Ga?" class="Bool (strict)"() -> ("Value"=w169:bool)  [unwired: 2 in, 2 out]
              n209 = case shown="True" w169 {
                frame False {
                  w171 = FALSE ("Ga Active")
                  w170 = 0.0 ("Ga Flow 1")
                  n210 = call "set_Ga.vi"("Active"=w171, "GAMFC3"=w170, "GAMFC2"=w170, "GAMFC1"=w170, "Bubbler In"=w171, "H2 Dilute"=w171, "Run"=w171, "Remote"=w171) -> ()  [unwired: 8 out]
                }
                frame True {
                  w175 = TRUE ("Ga Active")
                  n211 = property on="GAMFC3 var" class="DigNum (strict)"() -> ("Value"=w172:dbl)  [unwired: 2 in, 2 out]
                  n212 = property on="GAMFC2 var" class="DigNum (strict)"() -> ("Value"=w173:dbl)  [unwired: 2 in, 2 out]
                  n213 = property on="GAMFC1 var" class="DigNum (strict)"() -> ("Value"=w174:dbl)  [unwired: 2 in, 2 out]
                  n214 = property on="Prep-Ga var" class="Bool (strict)"() -> ("Value"=w176:bool)  [unwired: 2 in, 2 out]
                  n215 = property on="Run Ga" class="Bool (strict)"() -> ("Value"=w177:bool)  [unwired: 2 in, 2 out]
                  n216 = And(x=w176, y=w177) -> (x .and. y?=w179:bool)
                  n217 = property on="Ga Dilution" class="Bool (strict)"() -> ("Value"=w178:bool)  [unwired: 2 in, 2 out]
                  n218 = call "set_Ga.vi"("Active"=w175, "GAMFC3"=w172, "GAMFC2"=w173, "GAMFC1"=w174, "Bubbler In"=w175, "H2 Dilute"=w178, "Run"=w179, "Remote"=w175) -> ()  [unwired: 8 in]
                }
              }
            }
            frame True {
            }
          }
        }
        frame #2 {
          n219 = case shown="False" w180 {
            frame False {
              n220 = property on="In?" class="Bool (strict)"() -> ("Value"=w181:bool)  [unwired: 2 in, 2 out]
              n221 = case shown="True" w181 {
                frame False {
                  w183 = FALSE ("In Remote")
                  n222 = call "set_In.vi"("INMFC1"=0.0 ("Indium Flow"), "Remote"=w183, "Run"=w183, "Bubbler In"=w183, "Active"=w183) -> ()  [unwired: 5 out]
                }
                frame True {
                  w188 = TRUE ("In Run")
                  n223 = property on="Run In" class="Bool (strict)"() -> ("Value"=w185:bool)  [unwired: 2 in, 2 out]
                  n224 = property on="Prep In" class="Bool (strict)"() -> ("Value"=w186:bool)  [unwired: 2 in, 2 out]
                  n225 = And(x=w186, y=w185) -> (x .and. y?=w184:bool)
                  n226 = property on="In Flow" class="DigNum (strict)"() -> ("Value"=w187:dbl)  [unwired: 2 in, 2 out]
                  n227 = call "set_In.vi"("INMFC1"=w187, "Run"=w184, "Bubbler In"=w188, "Active"=w188) -> ()  [unwired: 1 in, 5 out]
                }
              }
            }
            frame True {
            }
          }
        }
        frame #3 {
          n228 = case shown="False" w189 {
            frame False {
              n229 = property on="PH3?" class="Bool (strict)"() -> ("Value"=w190:bool)  [unwired: 2 in, 2 out]
              n230 = case shown="True" w190 {
                frame False {
                  w191 = FALSE ("P_Gas Active")
                  n231 = call "set_P_gas.vi"("Run"=w191, "Gas In"=w191, "Active"=w191, "P_Gas Remote"=w191, "H2 Flush"=w191, "P_Gas Flow"=0.0) -> ()
                }
                frame True {
                  w197 = TRUE ("P_Gas Active")
                  n232 = property on="P Flow" class="DigNum (strict)"() -> ("Value"=w196:dbl)  [unwired: 2 in, 2 out]
                  n233 = property on="Prep P" class="Bool (strict)"() -> ("Value"=w195:bool)  [unwired: 2 in, 2 out]
                  n234 = property on="Run P" class="Bool (strict)"() -> ("Value"=w194:bool)  [unwired: 2 in, 2 out]
                  n235 = And(x=w195, y=w194) -> (x .and. y?=w193:bool)
                  n236 = call "set_P_gas.vi"("Active"=w197, "P_Gas Remote"=w193, "H2 Flush"=w197, "P_Gas Flow"=w196) -> ()  [unwired: 2 in]
                }
              }
            }
            frame True {
            }
          }
        }
        frame #4 {
          n237 = case shown="False" w198 {
            frame False {
              n238 = property on="AsH3?" class="Bool (strict)"() -> ("Value"=w199:bool)  [unwired: 2 in, 2 out]
              n239 = case shown="True" w199 {
                frame False {
                  w200 = FALSE ("As_Gas Active")
                  n240 = call "set_As_gas.vi"("Active"=w200, "As_Gas Flow"=0.0, "Gas In"=w200, "H2 Flush"=w200, "Run"=w200, "Remote"=w200) -> ()  [unwired: 10 in]
                }
                frame True {
                  w206 = TRUE ("As_Gas Active")
                  n241 = property on="Prep As" class="Bool (strict)"() -> ("Value"=w203:bool)  [unwired: 2 in, 2 out]
                  n242 = property on="Run As" class="Bool (strict)"() -> ("Value"=w204:bool)  [unwired: 2 in, 2 out]
                  n243 = property on="AsH3 Flow" class="DigNum (strict)"() -> ("Value"=w205:dbl)  [unwired: 2 in, 2 out]
                  n244 = And(x=w203, y=w204) -> (x .and. y?=w202:bool)
                  n245 = call "set_As_gas.vi"("Active"=w206, "As_Gas Flow"=w205, "Gas In"=w206, "Run"=w202) -> ()  [unwired: 12 in]
                }
              }
            }
            frame True {
            }
          }
        }
      }
    }
    frame "Run" {
      n246 = stacked-sequence {
        tunnel: w210 -> [_ w215 _ _]
        tunnel: w207 -> [w212 _ _ w269]
        tunnel: [_ _ _ w268] -> w209
        tunnel: w208 -> [_ _ _ w270]
        frame #0 {
          n247 = call "Get_Argument.vi"("Argument"="run_started", "Argument List"=w212) -> ("Enabled"=w211:bool)
          n248 = local write "run started"(w211) -> ()
        }
        frame #1 {
          n249 = property on="prep_time" class="DigNum (strict)"() -> ("Value"=w216:dbl)  [unwired: 2 in, 2 out]
          n250 = Greater Or Equal?(x=w215, y=w216) -> (x >= y?=w214:bool)
          n251 = local write "prep_done"(w214) -> ()
        }
        frame #2 {
          n252 = local read "run started"() -> (w218:bool)
          n253 = Not(x=w218) -> (.not. x?=w217:bool)
          n254 = stacked-sequence {
            tunnel: w217 -> [w220 w224 w233 w242 w251 w260]
            frame #0 {
              n255 = case shown="True" w220 {
                tunnel: ["run: " "pre-run: "] -> w219
                frame False {
                }
                frame True {
                }
              }
              n256 = property on="Status Out" class="Str"("Value"=w219) -> ()  [unwired: 2 in, 2 out]
            }
            frame #1 {
              n257 = property on="Status Out" class="Str"() -> ("Value"=w230:string)  [unwired: 2 in, 2 out]
              n258 = property on="Al?" class="Bool (strict)"() -> ("Value"=w231:bool)  [unwired: 2 in, 2 out]
              n259 = property on="Run Al" class="Bool (strict)"() -> ("Value"=w223:bool)  [unwired: 2 in, 2 out]
              n260 = property on="Prep Al" class="Bool (strict)"() -> ("Value"=w225:bool)  [unwired: 2 in, 2 out]
              n261 = call "flow_strings.vi"("string in"=w230, "is first in?"=TRUE, "use source?"=w231, "name"="Al", "run source?"=w223, "prep source?"=w225, "is prep?"=w224) -> ("string out"=w229:string, "is first out?"=w228:bool)
              n262 = property on="Status Out" class="Str"("Value"=w229) -> ()  [unwired: 2 in, 2 out]
              n263 = property on="first" class="Bool (strict)"("Value"=w228) -> ()  [unwired: 2 in, 2 out]
            }
            frame #2 {
              n264 = property on="first" class="Bool (strict)"() -> ("Value"=w236:bool)  [unwired: 2 in, 2 out]
              n265 = property on="Status Out" class="Str"() -> ("Value"=w239:string)  [unwired: 2 in, 2 out]
              n266 = property on="Ga?" class="Bool (strict)"() -> ("Value"=w237:bool)  [unwired: 2 in, 2 out]
              n267 = property on="Run Ga" class="Bool (strict)"() -> ("Value"=w232:bool)  [unwired: 2 in, 2 out]
              n268 = property on="Prep Ga" class="Bool (strict)"() -> ("Value"=w234:bool)  [unwired: 2 in, 2 out]
              n269 = call "flow_strings.vi"("string in"=w239, "is first in?"=w236, "use source?"=w237, "name"="Ga", "run source?"=w232, "prep source?"=w234, "is prep?"=w233) -> ("string out"=w240:string, "is first out?"=w235:bool)
              n270 = property on="Status Out" class="Str"("Value"=w240) -> ()  [unwired: 2 in, 2 out]
              n271 = property on="first" class="Bool (strict)"("Value"=w235) -> ()  [unwired: 2 in, 2 out]
            }
            frame #3 {
              n272 = property on="first" class="Bool (strict)"() -> ("Value"=w246:bool)  [unwired: 2 in, 2 out]
              n273 = property on="Status Out" class="Str"() -> ("Value"=w248:string)  [unwired: 2 in, 2 out]
              n274 = property on="In?" class="Bool (strict)"() -> ("Value"=w249:bool)  [unwired: 2 in, 2 out]
              n275 = property on="Run In" class="Bool (strict)"() -> ("Value"=w241:bool)  [unwired: 2 in, 2 out]
              n276 = property on="Prep In" class="Bool (strict)"() -> ("Value"=w243:bool)  [unwired: 2 in, 2 out]
              n277 = call "flow_strings.vi"("string in"=w248, "is first in?"=w246, "use source?"=w249, "name"="In", "run source?"=w241, "prep source?"=w243, "is prep?"=w242) -> ("string out"=w245:string, "is first out?"=w244:bool)
              n278 = property on="Status Out" class="Str"("Value"=w245) -> ()  [unwired: 2 in, 2 out]
              n279 = property on="first" class="Bool (strict)"("Value"=w244) -> ()  [unwired: 2 in, 2 out]
            }
            frame #4 {
              n280 = property on="first" class="Bool (strict)"() -> ("Value"=w254:bool)  [unwired: 2 in, 2 out]
              n281 = property on="Status Out" class="Str"() -> ("Value"=w256:string)  [unwired: 2 in, 2 out]
              n282 = property on="PH3?" class="Bool (strict)"() -> ("Value"=w257:bool)  [unwired: 2 in, 2 out]
              n283 = property on="Run P" class="Bool (strict)"() -> ("Value"=w250:bool)  [unwired: 2 in, 2 out]
              n284 = property on="Prep P" class="Bool (strict)"() -> ("Value"=w252:bool)  [unwired: 2 in, 2 out]
              n285 = call "flow_strings.vi"("string in"=w256, "is first in?"=w254, "use source?"=w257, "name"="P", "run source?"=w250, "prep source?"=w252, "is prep?"=w251) -> ("string out"=w255:string, "is first out?"=w253:bool)
              n286 = property on="Status Out" class="Str"("Value"=w255) -> ()  [unwired: 2 in, 2 out]
              n287 = property on="first" class="Bool (strict)"("Value"=w253) -> ()  [unwired: 2 in, 2 out]
            }
            frame #5 {
              n288 = property on="first" class="Bool (strict)"() -> ("Value"=w263:bool)  [unwired: 2 in, 2 out]
              n289 = property on="Status Out" class="Str"() -> ("Value"=w265:string)  [unwired: 2 in, 2 out]
              n290 = property on="AsH3?" class="Bool (strict)"() -> ("Value"=w266:bool)  [unwired: 2 in, 2 out]
              n291 = property on="Run As" class="Bool (strict)"() -> ("Value"=w259:bool)  [unwired: 2 in, 2 out]
              n292 = property on="Prep As" class="Bool (strict)"() -> ("Value"=w261:bool)  [unwired: 2 in, 2 out]
              n293 = call "flow_strings.vi"("string in"=w265, "is first in?"=w263, "use source?"=w266, "name"="As", "run source?"=w259, "prep source?"=w261, "is prep?"=w260) -> ("string out"=w262:string, "is first out?"=w264:bool)
              n294 = property on="Status Out" class="Str"("Value"=w262) -> ()  [unwired: 2 in, 2 out]
              n295 = property on="first" class="Bool (strict)"("Value"=w264) -> ()  [unwired: 2 in, 2 out]
            }
          }
        }
        frame #3 {
          n296 = local read "run started"() -> (w273:bool)
          n297 = local read "prep_done"() -> (w271:bool)
          n298 = Not(x=w273) -> (.not. x?=w274:bool)
          n299 = And(x=w271, y=w274) -> (x .and. y?=w272:bool)
          n300 = stacked-sequence {
            tunnel: w272 -> [w278]
            tunnel: w270 -> [w277]
            tunnel: w269 -> [w276]
            tunnel: [w275] -> w268
            frame #0 {
              n301 = case shown="True" w278 {
                tunnel: w277 -> [_ w282]
                tunnel: w276 -> [w279 w281]
                tunnel: [w279 w280] -> w275
                frame False {
                }
                frame True {
                  n302 = stacked-sequence {
                    tunnel: w282 -> [w283 w290 w300 w307 w314 _]
                    tunnel: w281 -> [_ _ _ _ _ w322]
                    tunnel: [_ _ _ _ _ w321] -> w280
                    frame #0 {
                      n303 = case shown="False" w283 {
                        frame False {
                          n304 = property on="Al?" class="Bool (strict)"() -> ("Value"=w284:bool)  [unwired: 2 in, 2 out]
                          n305 = case shown="True" w284 {
                            frame False {
                              w285 = FALSE ("Al Active")
                              n306 = call "set_Al.vi"("ALMFC1"=0.0 ("Aluminum Flow"), "Remote"=w285, "Run"=w285, "Bubbler In"=w285, "Active"=w285) -> ()  [unwired: 5 out]
                            }
                            frame True {
                              w289 = TRUE ("Al Active")
                              n307 = property on="Al Flow" class="DigNum (strict)"() -> ("Value"=w288:dbl)  [unwired: 2 in, 2 out]
                              n308 = property on="Run Al" class="Bool (strict)"() -> ("Value"=w287:bool)  [unwired: 2 in, 2 out]
                              n309 = call "set_Al.vi"("ALMFC1"=w288, "Run"=w287, "Bubbler In"=w289, "Active"=w289) -> ()  [unwired: 1 in, 5 out]
                            }
                          }
                        }
                        frame True {
                        }
                      }
                    }
                    frame #1 {
                      n310 = case shown="False" w290 {
                        frame False {
                          n311 = property on="Ga?" class="Bool (strict)"() -> ("Value"=w291:bool)  [unwired: 2 in, 2 out]
                          n312 = case shown="True" w291 {
                            frame False {
                              w293 = FALSE ("Ga Active")
                              w292 = 0.0 ("Ga Flow 1")
                              n313 = call "set_Ga.vi"("Active"=w293, "GAMFC3"=w292, "GAMFC2"=w292, "GAMFC1"=w292, "Bubbler In"=w293, "H2 Dilute"=w293, "Run"=w293, "Remote"=w293) -> ()  [unwired: 8 out]
                            }
                            frame True {
                              w298 = TRUE ("Ga Active")
                              n314 = property on="GAMFC3 var" class="DigNum (strict)"() -> ("Value"=w294:dbl)  [unwired: 2 in, 2 out]
                              n315 = property on="Ga Dilution" class="Bool (strict)"() -> ("Value"=w297:bool)  [unwired: 2 in, 2 out]
                              n316 = property on="Run Ga" class="Bool (strict)"() -> ("Value"=w299:bool)  [unwired: 2 in, 2 out]
                              n317 = property on="GAMFC2 var" class="DigNum (strict)"() -> ("Value"=w295:dbl)  [unwired: 2 in, 2 out]
                              n318 = property on="GAMFC1 var" class="DigNum (strict)"() -> ("Value"=w296:dbl)  [unwired: 2 in, 2 out]
                              n319 = call "set_Ga.vi"("Active"=w298, "GAMFC3"=w294, "GAMFC2"=w295, "GAMFC1"=w296, "Bubbler In"=w298, "H2 Dilute"=w297, "Run"=w299, "Remote"=w298) -> ()  [unwired: 8 in]
                            }
                          }
                        }
                        frame True {
                        }
                      }
                    }
                    frame #2 {
                      n320 = case shown="False" w300 {
                        frame False {
                          n321 = property on="In?" class="Bool (strict)"() -> ("Value"=w301:bool)  [unwired: 2 in, 2 out]
                          n322 = case shown="True" w301 {
                            frame False {
                              w303 = FALSE ("In Remote")
                              n323 = call "set_In.vi"("INMFC1"=0.0 ("Indium Flow"), "Remote"=w303, "Run"=w303, "Bubbler In"=w303, "Active"=w303) -> ()  [unwired: 5 out]
                            }
                            frame True {
                              w306 = TRUE ("In Run")
                              n324 = property on="Run In" class="Bool (strict)"() -> ("Value"=w304:bool)  [unwired: 2 in, 2 out]
                              n325 = property on="In Flow" class="DigNum (strict)"() -> ("Value"=w305:dbl)  [unwired: 2 in, 2 out]
                              n326 = call "set_In.vi"("INMFC1"=w305, "Run"=w304, "Bubbler In"=w306, "Active"=w306) -> ()  [unwired: 1 in, 5 out]
                            }
                          }
                        }
                        frame True {
                        }
                      }
                    }
                    frame #3 {
                      n327 = case shown="False" w307 {
                        frame False {
                          n328 = property on="PH3?" class="Bool (strict)"() -> ("Value"=w308:bool)  [unwired: 2 in, 2 out]
                          n329 = case shown="True" w308 {
                            frame False {
                              w309 = FALSE ("P_Gas Active")
                              n330 = call "set_P_gas.vi"("Run"=w309, "Gas In"=w309, "Active"=w309, "P_Gas Remote"=w309, "H2 Flush"=w309, "P_Gas Flow"=0.0) -> ()
                            }
                            frame True {
                              w313 = TRUE ("P_Gas Active")
                              n331 = property on="P Flow" class="DigNum (strict)"() -> ("Value"=w312:dbl)  [unwired: 2 in, 2 out]
                              n332 = property on="Run P" class="Bool (strict)"() -> ("Value"=w311:bool)  [unwired: 2 in, 2 out]
                              n333 = call "set_P_gas.vi"("Active"=w313, "P_Gas Remote"=w311, "H2 Flush"=w313, "P_Gas Flow"=w312) -> ()  [unwired: 2 in]
                            }
                          }
                        }
                        frame True {
                        }
                      }
                    }
                    frame #4 {
                      n334 = case shown="False" w314 {
                        frame False {
                          n335 = property on="AsH3?" class="Bool (strict)"() -> ("Value"=w315:bool)  [unwired: 2 in, 2 out]
                          n336 = case shown="True" w315 {
                            frame False {
                              w316 = FALSE ("As_Gas Active")
                              n337 = call "set_As_gas.vi"("Active"=w316, "As_Gas Flow"=0.0, "Gas In"=w316, "H2 Flush"=w316, "Run"=w316, "Remote"=w316) -> ()  [unwired: 10 in]
                            }
                            frame True {
                              w319 = TRUE ("As_Gas Active")
                              n338 = property on="Run As" class="Bool (strict)"() -> ("Value"=w318:bool)  [unwired: 2 in, 2 out]
                              n339 = property on="AsH3 Flow" class="DigNum (strict)"() -> ("Value"=w320:dbl)  [unwired: 2 in, 2 out]
                              n340 = call "set_As_gas.vi"("Active"=w319, "As_Gas Flow"=w320, "Gas In"=w319, "Run"=w318) -> ()  [unwired: 12 in]
                            }
                          }
                        }
                        frame True {
                        }
                      }
                    }
                    frame #5 {
                      n341 = call "Set_Argument.vi"("Enable"=TRUE, "Argument"="run_started", "Argument List In"=w322) -> ("Argument List Out"=w321:string[])
                    }
                  }
                }
              }
            }
          }
        }
      }
    }
    frame "End" {
    }
    frame "Idle" {
    }
  }
  "Argument List Out" <- w10
